vi "SetUhpCaptureMode.vi"(0 "Camera Reference in":refnum<k24>, 1 "error in (no error)":errorcluster, 4 "UhpCaptureMode (Camera1 Camera2 Merge)":u8(ring) items=["Camera1", "Camera2", "Merge"]) -> (2 "Camera Reference out":refnum<k24>, 3 "error out":errorcluster)   [LabVIEW 2023]
uses:
  C:/Users/mech-mind/Downloads/LabView/MechEyeApiNet.dll
  MechEyeApiNet.dll
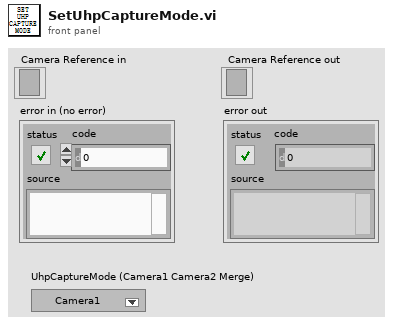
[diagram p1: front panel]
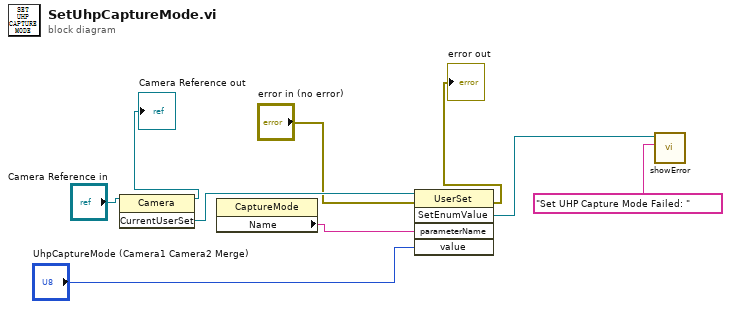
[diagram p0: block diagram]
diagram:
  n1 = invoke class="Camera" method="CurrentUserSet"(reference="Camera Reference in") -> (reference out=→"Camera Reference out":refnum<k24>, "CurrentUserSet"=w5:refnum<k24>)  [unwired: 2 in, 1 out]
  n2 = property class="CaptureMode"() -> ("Name"=w7:string)  [unwired: 2 in, 2 out]
  n3 = invoke class="UserSet" method="SetEnumValue"(reference=w5, error in="error in (no error)", "parameterName"=w7, "value"="UhpCaptureMode (Camera1 Camera2 Merge)") -> (error out=→"error out":errorcluster, "SetEnumValue"=w6:refnum<k24>)  [unwired: 1 in, 3 out]
  n4 = call "showError.vi"("String"="Set UHP Capture Mode Failed: ", "ErrorStatus Refnum in"=w6) -> ()  [unwired: 10 in]
